vi "Archive.vi"(8 "error in":errorcluster, 11 "Archive Data":T1) -> (0 "error out":errorcluster, 3 "archive name out":path)   [LabVIEW 2019, in "Archivist.lvclass"]
uses:
  Archivist.lvclass
  Settings/Dot Settings/Dot Settings.lvclass
  Settings/Setting Database/Typedefs/PublicEvents--Setting Database.DotsUpdated.ctl
  Settings/Setting Database/Setting Database.lvclass
  Settings/Funnel Settings/Funnel Settings.lvclass
  Settings/Setting Database/Typedefs/PublicEvents--Setting Database.FunnelsUpdated.ctl
  Settings/Rectangle Settings/Rectangle Settings.lvclass
  Settings/Setting Database/Typedefs/PublicEvents--Setting Database.RectanglesUpdated.ctl
  Settings/Path Settings/Path Settings.lvclass
  Settings/Setting Database/Typedefs/PublicEvents--Setting Database.PathsUpdated.ctl
  ArchiveData.ctl
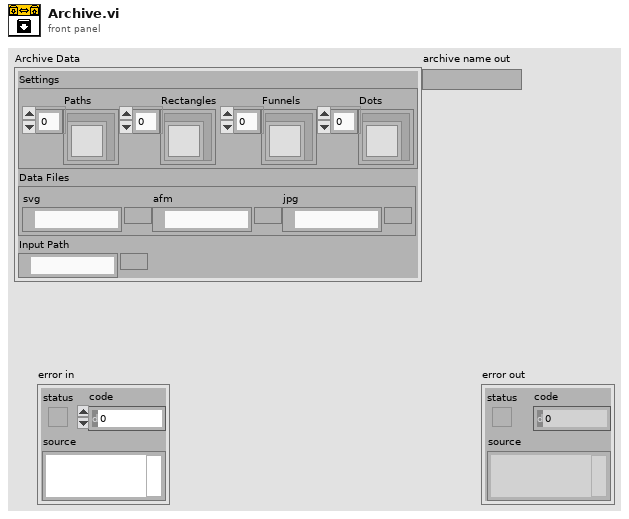
[diagram p1: front panel]
types:
  T1 = typedef "Archivist.lvclass/ArchiveData.ctl" = cluster{"Settings":cluster{"Paths":T2, "Rectangles":T3, "Funnels":T4, "Dots":T5}, "Data Files":cluster{"svg":path, "afm":path, "jpg":path}, "Input Path":path}
  T2 = typedef "Setting Database.lvclass/PublicEvents--Setting Database.PathsUpdated.ctl" = refnum<class "Path Settings.lvclass">[]
  T3 = typedef "Setting Database.lvclass/PublicEvents--Setting Database.RectanglesUpdated.ctl" = refnum<class "Rectangle Settings.lvclass">[]
  T4 = typedef "Setting Database.lvclass/PublicEvents--Setting Database.FunnelsUpdated.ctl" = refnum<class "Funnel Settings.lvclass">[]
  T5 = typedef "Setting Database.lvclass/PublicEvents--Setting Database.DotsUpdated.ctl" = refnum<class "Dot Settings.lvclass">[]
  T6 = cluster{"Paths":T2, "Rectangles":T3, "Funnels":T4, "Dots":T5}
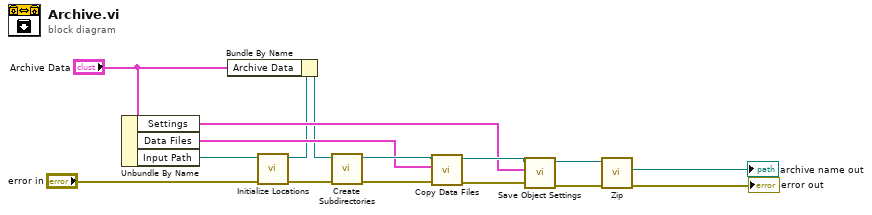
[diagram p0: block diagram]
diagram:
  n1 = Unbundle By Name("Archive Data") -> ("Settings"=w4:T6, "Data Files"=w5:cluster{"svg":path, "afm":path, "jpg":path}, "Input Path"=w6:path)
  n2 = call "Initialize Locations.vi"("error in"="error in", "Save Location"=w6) -> ("error out"=w14:errorcluster, "Archivist out"=w3:refnum<class "Archivist.lvclass">)  [unwired: 8 in]
  n3 = Bundle By Name(cluster=w3, "Archive Data"="Archive Data") -> (w2:refnum<class "Archivist.lvclass">)
  n4 = call "Create Subdirectories.vi"("error in"=w14, "Archivist in"=w2) -> ("error out"=w13:errorcluster, "Archivist out"=w16:refnum<class "Archivist.lvclass">)  [unwired: 8 in]
  n5 = call "Copy Data Files.vi"("error in"=w13, "Data Files"=w5, "Archivist in"=w16) -> ("error out"=w12:errorcluster, "Archivist out"=w15:refnum<class "Archivist.lvclass">)  [unwired: 7 in]
  n6 = call "Save Object Settings.vi"("error in"=w12, "Settings"=w4, "Archivist in"=w15) -> ("error out"=w10:errorcluster, "Archivist out"=w11:refnum<class "Archivist.lvclass">)  [unwired: 7 in]
  n7 = call "Zip.vi"("error in"=w10, "Archivist in"=w11) -> ("error out"=→"error out":errorcluster, "archive name out"=→"archive name out":path)  [unwired: 7 in, 1 out]
